vi "OAT Demodulation Initial Phase and CIC States.vi"(6 "CIC filter settings":T1={"interpolation/decimation factor"=2, "stages"=2, "lag"=1}, 7 "num of orders":i32, 8 "reset? (True)":bool=TRUE, 9 "CIC Image in":dbl[][](array[numeric]), 10 "CIC Real in":dbl[][](array[numeric]), 11 "start phase in":dbl[](array[numeric]) format="%.2f") -> (1 "CIC Image":dbl[][](array[numeric]), 2 "CIC Real":dbl[][](array[numeric]), 3 "start phase out":dbl[](array[numeric]) format="%.2f")   [LabVIEW 2017, in "SoundVib_Resampling.lvlib"]
uses:
  <vilib>/addons/Sound and Vibration/Order Analysis/Resample Order Tracking/SoundVib_Resampling.lvlib
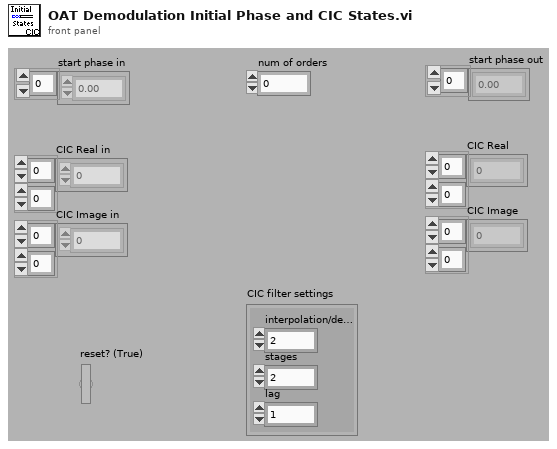
[diagram p1: front panel]
types:
  T1 = cluster{"interpolation/decimation factor":i32, "stages":i32, "lag":i32}
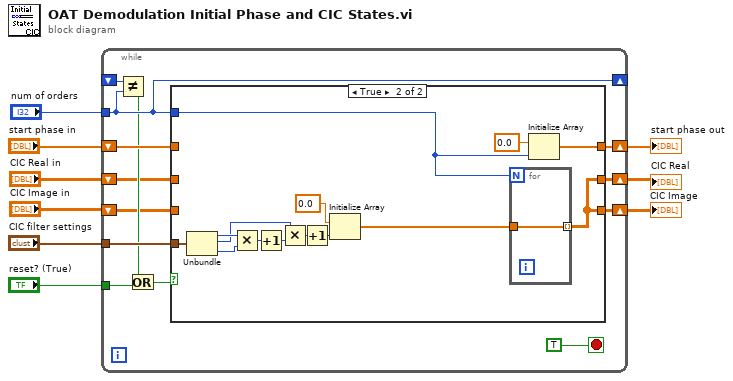
[diagram p0: block diagram]
diagram:
  n1 = while {
    tunnel: "reset? (True)" -> [w16]
    tunnel: "CIC filter settings" -> [w20]
    shift-right: [w17] -> _
    shift-left: _ -> [w18]
    tunnel: "num of orders" -> [w17]
    shift-right: [w13] -> w4
    shift-left: "CIC Real in" -> [w11]
    shift-right: [w12] -> w3
    shift-left: "CIC Image in" -> [w10]
    shift-right: [w22] -> w8
    shift-left: "start phase in" -> [w21]
    stop <- TRUE stop-if-true
    n2 = Not Equal?(x=w18, y=w17) -> (x != y?=w15:bool)
    n3 = Or(x=w15, y=w16) -> (x .or. y?=w14:bool)
    n4 = case shown="True" w14 {
      tunnel: [w25 w38] -> w22
      tunnel: w21 -> [w25 _]
      tunnel: w20 -> [_ w37]
      tunnel: w17 -> [_ w27]
      tunnel: [w24 w28] -> w13
      tunnel: [w23 w28] -> w12
      tunnel: w11 -> [w24 _]
      tunnel: w10 -> [w23 _]
      frame False {
      }
      frame True {
        n5 = Unbundle(w37) -> ("interpolation/decimation factor"=w35:i32, "stages"=w31:i32, "lag"=w34:i32)
        n6 = Multiply(x=w35, y=w34) -> (x*y=w33:i32)
        n7 = Increment(x=w33) -> (x+1=w32:i32)
        n8 = Multiply(x=w31, y=w32) -> (x*y=w30:i32)
        n9 = Increment(x=w30) -> (x+1=w29:i32)
        n10 = Initialize Array(0.0 ("Element Data"), w29) -> (w26:dbl[])
        n11 = for {
          N: w27 -> [_]
          tunnel: [w40] -> w28 mode=indexing
          tunnel: w26 -> [w40]
        }
        n12 = Initialize Array(0.0 ("Element Data"), w27) -> (w38:dbl[])
      }
    }
  }
  "start phase out" <- w8
  "CIC Real" <- w4
  "CIC Image" <- w3
